vi "U6 Stream Example LJ_swSLEEP.vi"() -> ()   [LabVIEW 2021]
panel:
  in  "Binary":bool
  in  "AIN Range":u16(ring) items=["LJ_rgBIP10V", "LJ_rgBIP1V", "LJ_rgBIPP1V", "LJ_rgBIPP01V"]
  in  "Scan List (-)":u8[](array[numeric])=[199, 199, 199, 199, 199, 199, 199, 199]
  in  "Resolution Index":u8
  out "Waveform Graph":dbl[][](graph)
  out "# Skipped Scans":i32
  in  "Simulated Processing Delay [ms]":u32
  out "UD Backlog [%]":dbl format="%.2f"
  in  "Scan List (+)":u8[](array[numeric])=[0, 1, 2, 3]
  out "Actual Scan Rate (Hz)":dbl=1000.0 format="%.3f"
  out "ms Per Loop":u32
  out "U3 Backlog [%]":dbl format="%.2f"
  out "Scans Retrieved Sec (measured)":dbl format="%.2f"
  out "# Scans Read":i32
  out "# of iterations":i32
  out "Data":dbl[][](array[numeric]) format="%.6f"
  in  "Scan Rate (Hz)":dbl=1000.0 format="%.3f"
  in  "Data File Extension":string="dat"
  out "Current Data File":path
  in  "Data File Prefix":string="data"
  in  "Write To File":bool
  in  "FirstFound":bool=TRUE
  in  "stop":bool
  in  "Address":string="1"
  out "Error Message":string
  # "Streams using the SLEEP wait mode."
  # "The actual scans/sec is controlled\nby hardware and is known.  This\n\"measured\" suggests the rate at\nwhich data is being retreived."
  # "0=Auto"
  # "(for all channels)"
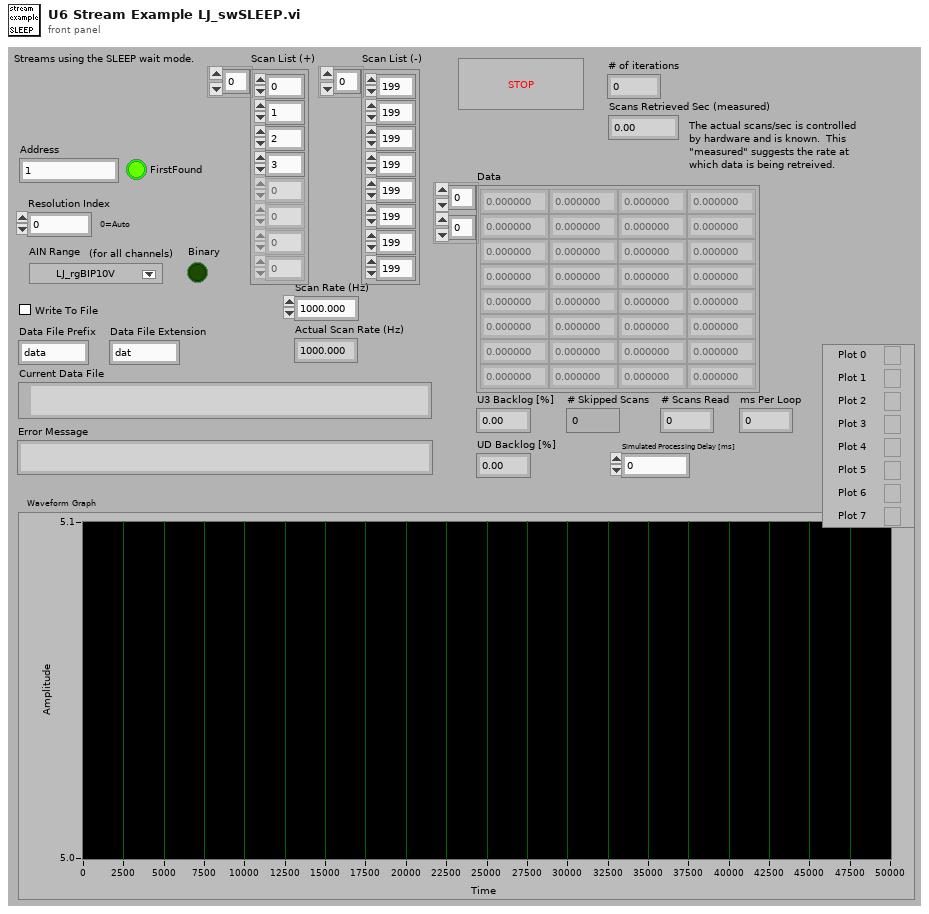
[diagram p1: front panel]
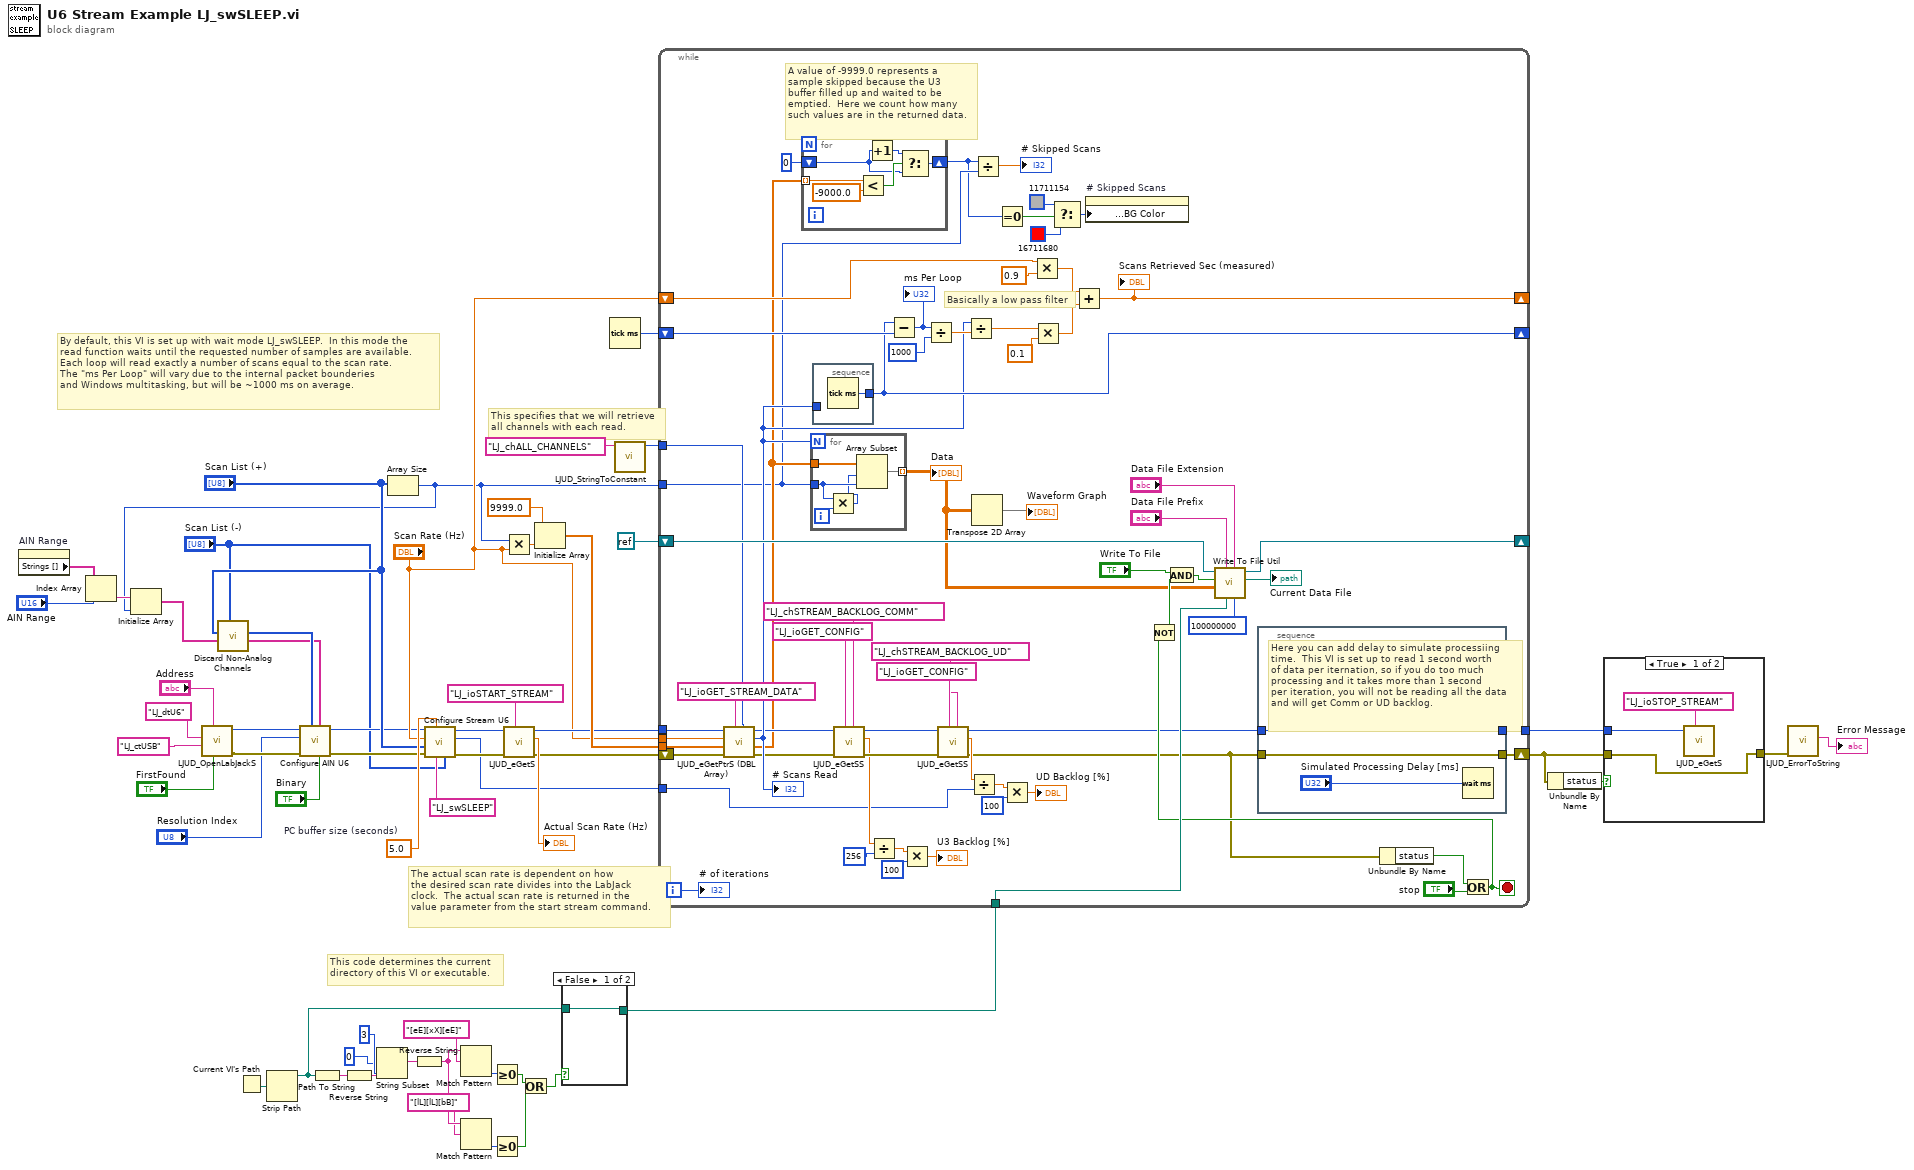
[diagram p0: block diagram]
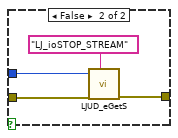
[diagram p2: hidden frame]
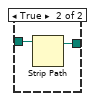
[diagram p3: hidden frame]
diagram:
  w27 = 5.0  # PC buffer size (seconds)
  # "This specifies that we will retrieve\nall channels with each read."
  # "The actual scan rate is dependent on how\nthe desired scan rate divides into the LabJack\nclock.  The actual scan rate is returned in the\nvalue parameter from the start stream command."
  # "By default, this VI is set up with wait mode LJ_swSLEEP.  In this mode the\nread function waits until the requested number of samples are available.\nEach loop will read exactly a number of scans equal to the scan rate.\nThe \"ms Per Loop\" will vary due to the internal packet bounderies\nand Windows multitasking, but will be ~1000 ms on average."
  # "This code determines the current\ndirectory of this VI or executable."
  n1 = property on="AIN Range" class="Ring (strict)"() -> ("Strings []"=w7:string[])  [unwired: 2 in, 2 out]
  n2 = Index Array(array=w7, index="AIN Range") -> (element=w5:string)
  n3 = call "LJUD_OpenLabJackS.vi"("FirstFound"="FirstFound", "Address"="Address", "ConnectionType"="LJ_ctUSB", "DeviceType"="LJ_dtU6") -> ("error out"=w11:errorcluster, "Handle"=w12:i32)  [unwired: 5 in, 1 out]
  n4 = Current VI's Path() -> (path=w54:path)
  n5 = Strip Path(path=w54) -> (stripped path=w46:path)  [unwired: 1 out]
  n6 = Path To String(path=w46) -> (string=w53:string)
  n7 = Reverse String(1:w53) -> (0:w52:string)
  n8 = String Subset(string=w52, offset (0)=0, length (rest)=3 ("length")) -> (substring=w49:string)
  n9 = Array Size(array="Scan List (+)") -> (size(s)=w4:i32)
  n10 = Initialize Array(w5, w4) -> (w3:string[])
  n11 = call "Discard Non-Analog Channels.vi"("Channels In (-)"="Scan List (-)", "Ranges In"=w3, "Channels In"="Scan List (+)") -> ("Ranges Out"=w9:string[], "Channels Out"=w10:i32[])  [unwired: 5 in, 2 out]
  n12 = call "Configure AIN U6.vi"("Binary"="Binary", "Ranges"=w9, "Positive Channels"=w10, "error in"=w11, "Resolution"="Resolution Index", "Handle In"=w12) -> ("error out"=w14:errorcluster, "Handle Out"=w13:i32)  [unwired: 4 in]
  n13 = Reverse String(1:w49) -> (0:w45:string)
  n14 = call "Configure Stream U6.vi"("Scan List (-)"="Scan List (-)", "Wait Mode"="LJ_swSLEEP" ("Wait Mode (2)"), "PC buffer size (seconds)"=w27, "error in"=w14, "Scan List (+)"="Scan List (+)", "Scan Rate (Hz)"="Scan Rate (Hz)", "Handle In"=w13) -> ("error out"=w36:errorcluster, "PC buffer size (samples)"=w18:i32, "Handle Out"=w37:i32)  [unwired: 2 in]
  n15 = Match Pattern(string=w45, regular expression="[eE][xX][eE]") -> (offset past match=w47:i32)  [unwired: 1 in, 3 out]
  n16 = Match Pattern(string=w45, regular expression="[lL][lL][bB]") -> (offset past match=w42:i32)  [unwired: 1 in, 3 out]
  n17 = Greater Or Equal To 0?(x=w47) -> (x >= 0?=w43:bool)
  n18 = Greater Or Equal To 0?(x=w42) -> (x >= 0?=w41:bool)
  n19 = Multiply(x=w4, y="Scan Rate (Hz)") -> (x*y=w35:dbl)
  n20 = call "LJUD_eGetS.vi"("IOType"="LJ_ioSTART_STREAM", "error in"=w36, "Handle In"=w37) -> ("error out"=w20:errorcluster, "Value Read"=→"Actual Scan Rate (Hz)":dbl, "Handle Out"=w25:i32)  [unwired: 6 in]
  n21 = Or(x=w43, y=w41) -> (x .or. y?=w40:bool)
  n22 = Initialize Array(9999.0, w35) -> (w33:dbl[])
  n23 = case shown="False" w40 {
    tunnel: w46 -> [w58 w60]
    tunnel: [w58 w59] -> w39
    frame False {
    }
    frame True {
      n24 = Strip Path(path=w60) -> (stripped path=w59:path)  [unwired: 1 out]
    }
  }
  n25 = Tick Count (ms)() -> (millisecond timer value=w28:u32)
  n26 = call "LJUD_StringToConstant.vi"("String"="LJ_chALL_CHANNELS") -> ("Constant Number"=w21:i32)  [unwired: 9 in, 1 out]
  n27 = while {
    tunnel: w18 -> [w79]
    shift-left: w20 -> [w87]
    shift-right: [w75] -> w19
    tunnel: w21 -> [w92]
    shift-left: "Scan Rate (Hz)" -> [w100]
    shift-right: [w97] -> _
    shift-left: w28 -> [w109]
    shift-right: [w106] -> _
    tunnel: [w73] -> w31
    tunnel: w4 -> [w70]
    tunnel: w33 -> [w112]
    tunnel: "Scan Rate (Hz)" -> [w111]
    tunnel: w39 -> [w116]
    shift-left: refnum<k0> refnum -> [w122]
    shift-right: [w121] -> _
    tunnel: w25 -> [w114]
    i -> [w110]
    stop <- w115 stop-if-true
    # "A value of -9999.0 represents a\nsample skipped because the U3\nbuffer filled up and waited to be\nemptied.  Here we count how many\nsuch values are in the returned data."
    # "Basically a low pass filter"
    n28 = call "LJUD_eGetPtrS (DBL Array).vi"("Channel"=w92, "IOType"="LJ_ioGET_STREAM_DATA", "error in"=w87, "DBL Array Write"=w112, "Value"=w111, "Handle In"=w114) -> ("error out"=w95:errorcluster, "DBL Array Read"=w72:dbl[], "Value"=w104:i32, "Handle Out"=w96:i32)  [unwired: 2 in]
    "# Scans Read" <- w104
    n29 = for {
      shift-right: [w127] -> w66
      shift-left: 0 -> [w128]
      tunnel: w72 -> [w131] mode=indexing
      n30 = Less?(x=w131, y=-9000.0) -> (x < y?=w129:bool)
      n31 = Increment(x=w128) -> (x+1=w132:i32)
      n32 = Select(t=w132, s=w129, f=w128) -> (s? t:f=w127:i32)
    }
    n33 = for {
      N: w104 -> [_]
      tunnel: w72 -> [w141]
      tunnel: w70 -> [w140]
      tunnel: [w137] -> w62 mode=indexing
      i -> [w139]
      n34 = Multiply(x=w140, y=w139) -> (x*y=w138:i32)
      n35 = Array Subset(array=w141, index=w138, length=w140) -> (w137:dbl[])
    }
    "Data" <- w62
    n36 = stacked-sequence {
      tunnel: w104 -> [_]
      tunnel: [w136] -> w106
      frame #0 {
        n37 = Tick Count (ms)() -> (millisecond timer value=w136:u32)
      }
    }
    n38 = call "LJUD_eGetSS.vi"("Channel"="LJ_chSTREAM_BACKLOG_COMM", "IOType"="LJ_ioGET_CONFIG", "error in"=w95, "Handle In"=w96) -> ("error out"=w88:errorcluster, "Value Read"=w83:dbl, "Handle Out"=w89:i32)  [unwired: 5 in]
    n39 = Divide(x=w83, y=256) -> (x/y=w86:dbl)
    n40 = Subtract(x=w106, y=w109) -> (x-y=w108:u32)
    "ms Per Loop" <- w108
    n41 = Multiply(x=w86, y=100) -> (x*y=→"U3 Backlog [%]":dbl)
    n42 = Divide(x=w108, y=u32 1000) -> (x/y=w105:dbl)
    n43 = call "LJUD_eGetSS.vi"("Channel"="LJ_chSTREAM_BACKLOG_UD", "IOType"="LJ_ioGET_CONFIG", "error in"=w88, "Handle In"=w89) -> ("error out"=w76:errorcluster, "Value Read"=w78:dbl, "Handle Out"=w74:i32)  [unwired: 5 in]
    n44 = Divide(x=w104, y=w105) -> (x/y=w103:dbl)
    n45 = Divide(x=w78, y=w79) -> (x/y=w80:dbl)
    n46 = Transpose 2D Array(2D array=w62) -> (transposed array=→"Waveform Graph":dbl[][])
    n47 = Divide(x=w66, y=w70) -> (x/y=→"# Skipped Scans":dbl)
    n48 = Equal To 0?(x=w66) -> (x = 0?=w65:bool)
    n49 = Multiply(x=w80, y=100) -> (x*y=→"UD Backlog [%]":dbl)
    n50 = Multiply(x=w100, y=0.9) -> (x*y=w99:dbl)
    n51 = Multiply(x=w103, y=0.1) -> (x*y=w98:dbl)
    n52 = Select(t=u32 11711154, s=w65, f=u32 16711680) -> (s? t:f=w64:u32)
    n53 = Add(x=w99, y=w98) -> (x+y=w97:dbl)
    "Scans Retrieved Sec (measured)" <- w97
    n54 = property on="# Skipped Scans" class="DigNum (strict)"("Numeric Text.Text Colors:BG Color"=w64) -> ()  [unwired: 2 in, 2 out]
    n55 = stacked-sequence {
      tunnel: w76 -> [w135]
      tunnel: [w135] -> w75
      tunnel: w74 -> [w134]
      tunnel: [w134] -> w73
      frame #0 {
        # "Here you can add delay to simulate processiing\ntime.  This VI is set up to read 1 second worth\nof data per iternation, so if you do too much\nprocessing and it takes more than 1 second\nper iteration, you will not be reading all the data\nand will get Comm or UD backlog."
        n56 = Wait (ms)(milliseconds to wait="Simulated Processing Delay [ms]") -> ()  [unwired: 1 out]
      }
    }
    n57 = Unbundle By Name(w76) -> ("status"=w125:bool)
    n58 = Or(x=w125, y="stop") -> (x .or. y?=w115:bool)
    n59 = Not(x=w115) -> (.not. x?=w117:bool)
    n60 = And(x="Write To File", y=w117) -> (x .and. y?=w118:bool)
    n61 = call "Write To File Util.vi"("Maximum File Size (Bytes)"=100000000, "Data File Extension"="Data File Extension", "Working Directory"=w116, "Data File Prefix"="Data File Prefix", "Data"=w62, "Write To File"=w118, "File Refnum In"=w122) -> ("Current Data File"=→"Current Data File":path, "File Refnum Out"=w121:refnum<file>)  [unwired: 2 in, 1 out]
    "# of iterations" <- w110
  }
  n62 = Unbundle By Name(w19) -> ("status"=w23:bool)
  n63 = case shown="True" w23 {
    tunnel: w31 -> [w143 w147]
    tunnel: [w142 w146] -> w30
    tunnel: w19 -> [w142 w145]
    frame True {
      n64 = call "LJUD_eGetS.vi"("IOType"="LJ_ioSTOP_STREAM", "Handle In"=w143) -> ()  [unwired: 7 in, 3 out]
    }
    frame False {
      n65 = call "LJUD_eGetS.vi"("IOType"="LJ_ioSTOP_STREAM", "error in"=w145, "Handle In"=w147) -> ("error out"=w146:errorcluster)  [unwired: 6 in, 2 out]
    }
  }
  n66 = call "LJUD_ErrorToString.vi"("error in"=w30) -> ("String"=→"Error Message":string)  [unwired: 10 in]
